vi "Receive Data.vi"(8 "Error In":errorcluster, 11 "VISA resource name":refnum<visa-resource-name>) -> (0 "Error Out":errorcluster, 4 "output cluster":T1 {"Battery Level" scale=0.0..255.0})   [LabVIEW 2014]
uses:
  Controls/Controllers Clusters/Normal Operation Indicator Cluster.ctl
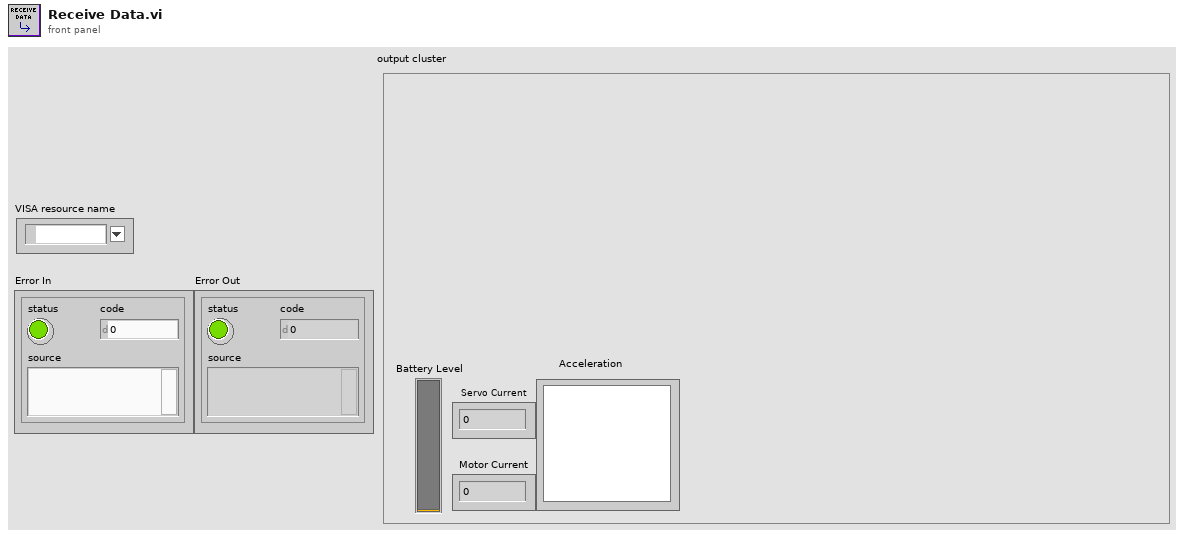
[diagram p1: front panel]
types:
  T1 = typedef "Normal Operation Indicator Cluster.ctl" = cluster{"Battery Level":u8, "Servo Current":dbl, "Motor Current":dbl, "Acceleration":cluster{"X":dbl, "Y":dbl}[]}
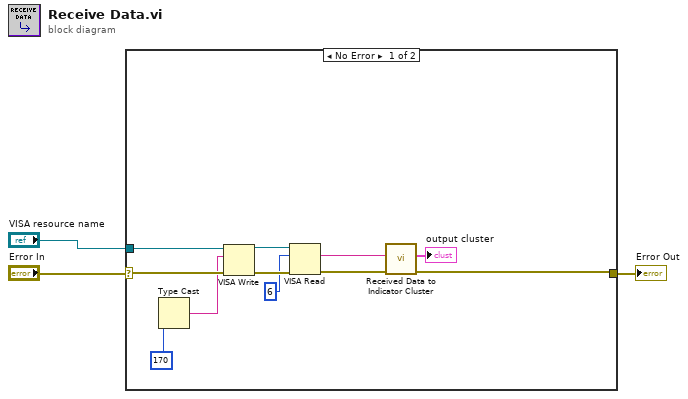
[diagram p0: block diagram]
diagram:
  n1 = case shown="No Error" "Error In" {
    selector: "Error In" -> [w10 w15]
    tunnel: [w6 w15] -> w2
    tunnel: "VISA resource name" -> [w9 _]
    frame No Error {
      n2 = Type Cast(x=u8 170) -> (*(type *) &x=w8:string)  [unwired: 1 in]
      n3 = VISA Write(VISA resource name=w9, write buffer=w8, error in (no error)=w10) -> (VISA resource name out=w12:refnum<visa-resource-name>, error out=w13:errorcluster)  [unwired: 1 out]
      n4 = VISA Read(VISA resource name=w12, byte count=u32 6, error in (no error)=w13) -> (read buffer=w5:string, error out=w7:errorcluster)  [unwired: 2 out]
      n5 = call "Received Data to Indicator Cluster.vi"("Error In"=w7, "Data"=w5) -> ("Error Out"=w6:errorcluster, "output cluster"=→"output cluster":T1)  [unwired: 8 in]
    }
    frame Error {
    }
  }
  "Error Out" <- w2
